vi "Get CAlex2.vi"(8 "error in (no error)":errorcluster, 11 "CAlexData2 in":refnum<class "CAlex2_Data.lvclass">) -> (0 "error out":errorcluster, 2 "CAlex2":refnum<class "CAlex2.lvclass">, 3 "CAlexData2 out":refnum<class "CAlex2_Data.lvclass">)   [LabVIEW 2016, in "CAlex2_Data.lvclass"]
uses:
  CAlex2_Data.lvclass
  Classes/CAlex2/CAlex2.lvclass
  CAlex2_Data.lvclass/CAlex2_Data.ctl
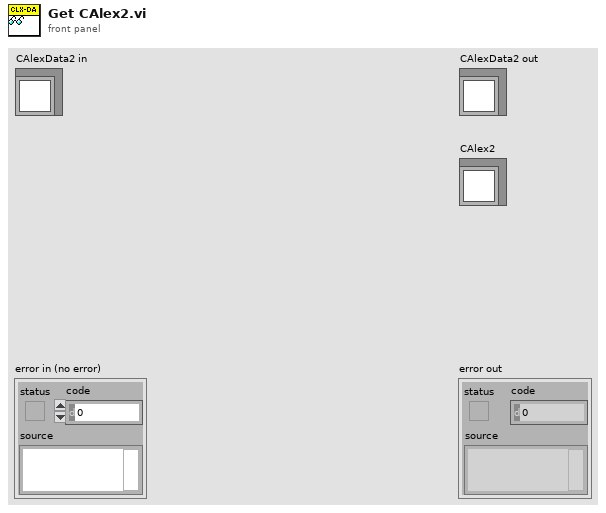
[diagram p1: front panel]
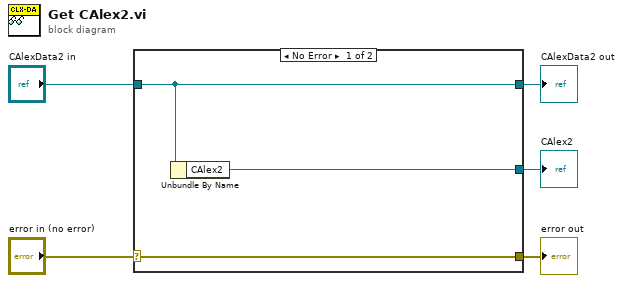
[diagram p0: block diagram]
diagram:
  n1 = case shown="No Error" "error in (no error)" {
    selector: "error in (no error)" -> [w8 w9]
    tunnel: [w8 w9] -> w4
    tunnel: [w7 w10] -> w2
    tunnel: "CAlexData2 in" -> [w7 w10]
    tunnel: [w6 _] -> w1
    frame No Error {
      n2 = Unbundle By Name(w7) -> ("CAlex2"=w6:refnum<class "CAlex2.lvclass">)
    }
    frame Error {
    }
  }
  "error out" <- w4
  "CAlexData2 out" <- w2
  "CAlex2" <- w1
